vi "海流计数据编码.vi"() -> (3 "发送的信息":string)   [LabVIEW 2016, in "数据传输系统-03.lvlib"]
panel:
  out "层数 2":string
  out "层数参数位置 2":i32
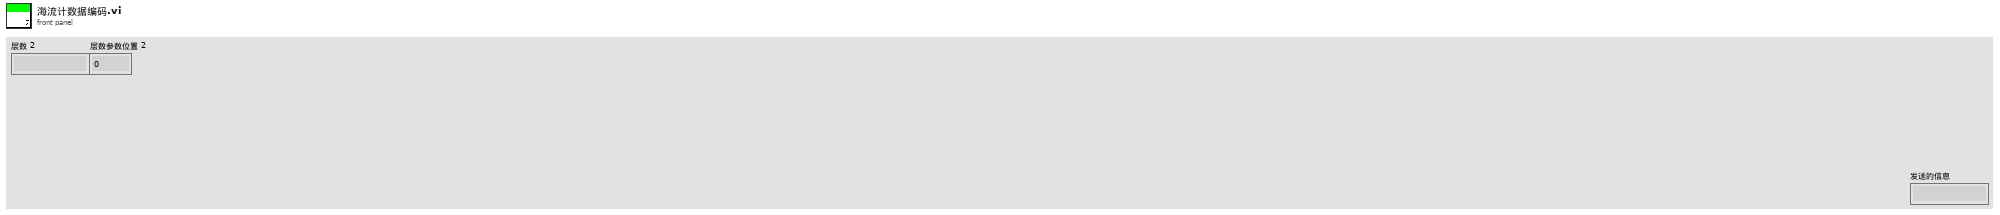
[diagram p1: front panel]
types:
  T1 = cluster{"CODMn":string, "CODCr":string, "DO":string, "铜":string, "PH":string, "氨氮":string, "比电导率":string, "水温":string, "COD":string, "浊度":string, "总氮":string, "总磷":string, "叶绿素a":string, "藻密度":string, "水位":string, "流速":string, "方向":string, "瞬时流量":string, "累积流量":string, "正累积流量":string, "负累积流量":string, "亚硝酸盐":string, "硫化物":string, "ORP":string, "铅":string, "镉":string, "锌":string, "镍":string, "锰":string, "汞":string, "气温":string, "气压":string, "风速":string, "风向":string, "空气温度":string, "相对湿度":string, "分钟雨量":string, "小时雨量":string, "日雨量":string, "累积雨量":string, "盐度":string, "磷酸盐":string, "硝氮":string, "氟化物":string, "挥发酚":string, "氯化物":string, "蓝绿藻":string, "余氯":string, "综合生物毒性":string, "艏向":string, "横摇":string, "纵摇":string, "分层标志":string, "层状态1":string, "层状态2":string, "水平平均流速":string, "流向":string, "北向流速分量":string, "东向流速分量":string, "垂直流速分量":string, "最大波高":string, "最大波周期":string, "1/10波高":string, "1/10波周期":string, "有效波高":string, "有效波周期":string, "平均波高":string, "平均波周期":string, "波向":string, "波个数":string, "水深":string, "X轴流速":string, "Y轴流速":string, "信号强度":string, "电压":string, "悬浮物":string}
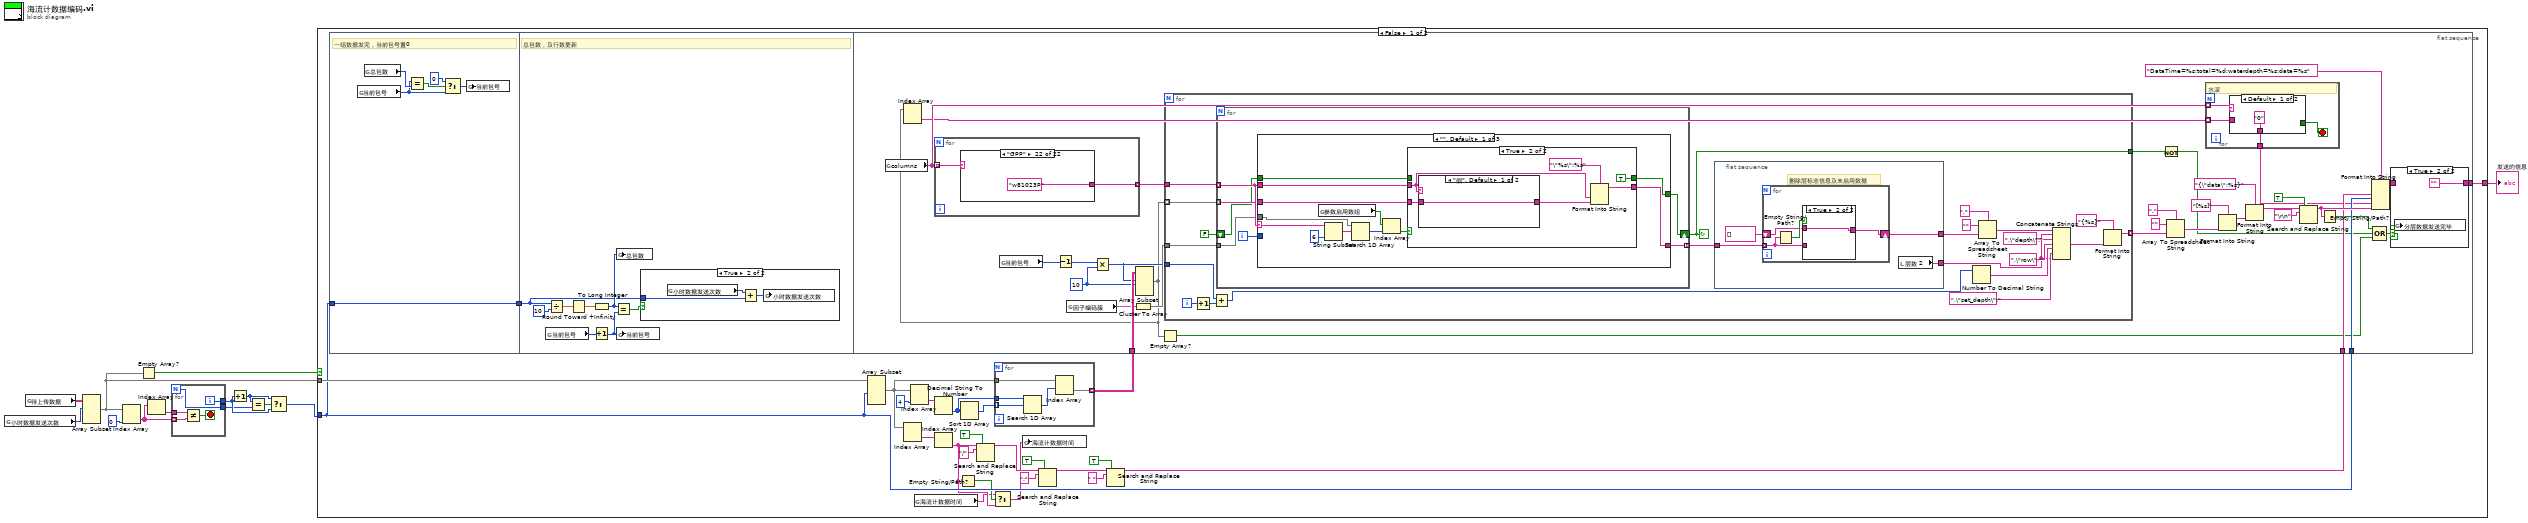
[diagram p0: block diagram]
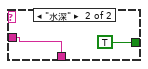
[diagram p3: hidden frame]
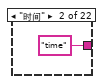
[diagram p6: hidden frame]
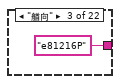
[diagram p7: hidden frame]
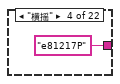
[diagram p8: hidden frame]
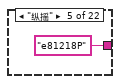
[diagram p9: hidden frame]
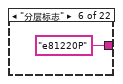
[diagram p10: hidden frame]
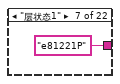
[diagram p11: hidden frame]
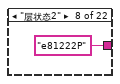
[diagram p12: hidden frame]
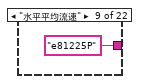
[diagram p13: hidden frame]
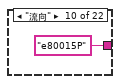
[diagram p14: hidden frame]
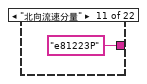
[diagram p15: hidden frame]
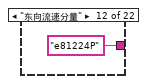
[diagram p16: hidden frame]
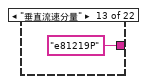
[diagram p17: hidden frame]
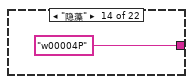
[diagram p18: hidden frame]
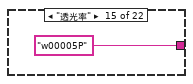
[diagram p19: hidden frame]
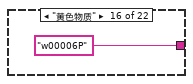
[diagram p20: hidden frame]
diagram:
  n1 = global read "全局 小时数据发送次数.vi" "小时数据发送次数"() -> (w13:i32)
  n2 = global read "全局 所有参数.vi" "待上传数据"() -> (w8:string[][])
  n3 = Array Subset(array=w8, index (row)=w13) -> (w6:string[][])  [unwired: 3 in]
  n4 = Index Array(array=w6, index (col)=0 ("禁用的索引 (列)")) -> (element=w11:string[])  [unwired: 1 in]
  n5 = Empty Array?(array=w6) -> (empty?=w7:bool)
  n6 = Index Array(array=w11) -> (element=w10:string)  [unwired: 1 in]
  n7 = for {
    N -> [w14]
    tunnel: w11 -> [w17] mode=indexing
    tunnel: w10 -> [w18]
    tunnel: [w15] -> w3
    tunnel: [w14] -> w2
    i -> [w15]
    stop <- w16 stop-if-true
    n8 = Not Equal?(x=w18, y=w17) -> (x != y?=w16:bool)
  }
  n9 = Increment(x=w3) -> (x+1=w4:i32)
  n10 = Equal?(x=w4, y=w2) -> (x = y?=w5:bool)
  n11 = Select(t=w4, s=w5, f=w3) -> (s? t:f=w1:i32)
  n12 = case shown="False" w7 {
    selector: w7 -> [_ w214]
    tunnel: w1 -> [w35 _]
    tunnel: w6 -> [w41 _]
    tunnel: [w19 _] -> w9
    frame False {
      n13 = flat-sequence {
        tunnel: w35 -> [w48]
        tunnel: [w48] -> w42
        tunnel: w42 -> [w54]
        tunnel: w37 -> [w97]
        tunnel: w35 -> [w77]
        tunnel: w20 -> [w76]
        tunnel: [w72] -> w19
        frame #0 {
          # "一组数据发完，当前包号置0"
          n14 = global read "全局 数据数组大小.vi" "当前包号"() -> (w51:i32)
          n15 = global read "全局 数据数组大小.vi" "总包数"() -> (w53:i32)
          n16 = Equal?(x=w51, y=w53) -> (x = y?=w52:bool)
          n17 = Select(t=0, s=w52, f=w51) -> (s? t:f=w49:i32)
          n18 = global write "全局 数据数组大小.vi" "当前包号"(w49) -> ()
        }
        frame #1 {
          # "总包数，及行数更新"
          n19 = global read "全局 数据数组大小.vi" "当前包号"() -> (w58:i32)
          n20 = Divide(x=w54, y=10) -> (x/y=w60:dbl)
          n21 = Round Toward +Infinity(x=w60) -> (ceil(x): smallest int >= x=w61:dbl)
          n22 = To Long Integer(number=w61) -> (32bit integer=w57:i32)
          n23 = Increment(x=w58) -> (x+1=w56:i32)
          n24 = Equal?(x=w57, y=w56) -> (x = y?=w55:bool)
          n25 = global write "全局 数据数组大小.vi" "总包数"(w57) -> ()
          n26 = global write "全局 数据数组大小.vi" "当前包号"(w56) -> ()
          n27 = case shown="True" w55 {
            tunnel: w54 -> [_ w63]
            frame False {
            }
            frame True {
              n28 = global read "全局 小时数据发送次数.vi" "小时数据发送次数"() -> (w64:i32)
              n29 = Add(x=w64, y=w63) -> (x+y=w62:i32)
              n30 = global write "全局 小时数据发送次数.vi" "小时数据发送次数"(w62) -> ()
            }
          }
        }
        frame #2 {
          w94 = 10 ("长度")
          n31 = global read "全局 所有参数.vi" "columns"() -> (w68:string[])
          n32 = for {
            tunnel: w68 -> [w109] mode=indexing
            tunnel: [w108] -> w91 mode=indexing
            n33 = case shown="\"GPP\"" w109 {
              tunnel: [_ "time" ("元素") "e81216P" "e81217P" "e81218P" "e81220P" "e81221P" "e81222P" "e81225P" "e80015P" "e81223P" "e81224P" "e81219P" "w00004P" "w00005P" "w00006P" "w00007P" "w01002P" "w01022P" "w81024P" "w81025P" "w81023P"] -> w108
              frame "", Default {
              }
              frame "时间" {
              }
              frame "艏向" {
              }
              frame "横摇" {
              }
              frame "纵摇" {
              }
              frame "分层标志" {
              }
              frame "层状态1" {
              }
              frame "层状态2" {
              }
              frame "水平平均流速" {
              }
              frame "流向" {
              }
              frame "北向流速分量" {
              }
              frame "东向流速分量" {
              }
              frame "垂直流速分量" {
              }
              frame "隐藻" {
              }
              frame "透光率" {
              }
              frame "黄色物质" {
              }
              frame "总藻" {
              }
              frame "盐度" {
              }
              frame "蓝绿藻" {
              }
              frame "Fv/Fm" {
              }
              frame "PAR" {
              }
              frame "GPP" {
              }
            }
          }
          n34 = global read "全局 数据数组大小.vi" "当前包号"() -> (w96:i32)
          n35 = Decrement(x=w96) -> (x-1=w95:i32)
          n36 = global read "断电保存全局.vi" "因子编码簇"() -> (w93:T1)
          n37 = Multiply(x=w95, y=w94) -> (x*y=w90:i32)
          n38 = Cluster To Array(cluster=w93) -> (array=w92:string[])
          n39 = Array Subset(array=w97, index (row)=w90, length (row)=w94) -> (w67:string[][])  [unwired: 2 in]
          n40 = Index Array(array=w67) -> (element=w66:string[])  [unwired: 2 in]
          n41 = Empty Array?(array=w67) -> (empty?=w69:bool)
          n42 = for {
            tunnel: w67 -> [w151] mode=indexing
            tunnel: w91 -> [w152]
            tunnel: [w147] -> w78 mode=indexing
            tunnel: w92 -> [w134]
            tunnel: [w132] -> w75
            tunnel: w90 -> [w131]
            i -> [w146]
            stop <- w132 continue-if-true
            n43 = Increment(x=w146) -> (x+1=w138:i32)
            n44 = Add(x=w131, y=w138) -> (x+y=w139:i32)
            n45 = for {
              tunnel: w152 -> [w170] mode=indexing
              tunnel: w151 -> [w169] mode=indexing
              tunnel: [w171] -> w137 mode=indexing
              tunnel: w134 -> [w167]
              shift-right: [w165] -> w132
              shift-left: FALSE -> [w166]
              i -> [w168]
              n46 = case shown="\"\", Default" w170 {
                selector: w170 -> [w175 _ _]
                tunnel: [w183 "" w212] -> w171
                tunnel: w170 -> [w182 w203 w211]
                tunnel: w169 -> [w181 w202 w207]
                tunnel: w168 -> [_ w201 _]
                tunnel: w167 -> [w180 _ _]
                tunnel: w166 -> [w176 w199 w205]
                tunnel: [w177 w199 w205] -> w165
                frame "", Default {
                  n47 = global read "断电保存全局.vi" "参数启用数组"() -> (w179:bool[])
                  n48 = String Subset(string=w175, length (rest)=6 ("长度（剩余）")) -> (substring=w173:string)  [unwired: 1 in]
                  n49 = Search 1D Array(1D array=w180, element=w173) -> (index of element=w178:i32)  [unwired: 1 in]
                  n50 = Index Array(array=w179, index=w178) -> (element=w172:bool)
                  n51 = case shown="True" w172 {
                    tunnel: ["" w190] -> w183
                    tunnel: w182 -> [_ w188]
                    tunnel: w181 -> [_ w187]
                    tunnel: [w184 TRUE] -> w177
                    tunnel: w176 -> [w184 _]
                    frame False {
                    }
                    frame True {
                      n52 = case shown="\"假\", Default" w188 {
                        tunnel: w187 -> [w192 w198]
                        tunnel: [w192 w193] -> w186
                        frame "假", Default {
                        }
                        frame "e81219P", "e81223P", "e81224P", "e81225P" {
                          n53 = Fract/Exp String To Number(string=w198) -> (number=w197:dbl)  [unwired: 3 in, 1 out]
                          n54 = Divide(x=w197, y=100.0) -> (x/y=w195:dbl)
                          n55 = Number To Fractional String(number=w195, precision (6)=i16 3 ("精度(6)")) -> (F-format string=w193:string)  [unwired: 2 in]
                        }
                      }
                      n56 = Format Into String(format string="\"%s\":%s" ("格式字符串"), w188, w186) -> (resulting string=w190:string)  [unwired: 2 in, 1 out]
                    }
                  }
                }
                frame "e81220P" {
                  n57 = Format Into String(format string="\"%s\":%s" ("格式字符串"), w203, w202) -> ()  [unwired: 2 in, 2 out]
                  "层数 2" <- w202
                  "层数参数位置 2" <- w201
                }
                frame "time" {
                  n58 = Search and Replace String(replace all?=TRUE ("替换全部？(F)"), input string=w207, search string="/" ("搜索字符串"), replace string="-" ("替换字符串(\"\")")) -> (result string=w206:string)  [unwired: 4 in, 3 out]
                  n59 = Format Into String(format string="\"%s\":\"%s\"" ("格式字符串"), w211, w206) -> (resulting string=w212:string)  [unwired: 2 in, 1 out]
                }
              }
            }
            n60 = flat-sequence {
              tunnel: w137 -> [w155]
              tunnel: [w156] -> w136
              tunnel: [w153] -> w135
              frame #0 {
                # "删除层标志信息及未启用数据"
                n61 = for {
                  tunnel: w155 -> [w157] mode=indexing
                  shift-right: [w158] -> w153
                  shift-left: string[] [] -> [w159]
                  n62 = Empty String/Path?(string/path=w157) -> (empty?=w160:bool)
                  n63 = case shown="True" w160 {
                    tunnel: [w161 w164] -> w158
                    tunnel: w159 -> [w163 w164]
                    tunnel: w157 -> [w162 _]
                    frame False {
                      n64 = Build Array (concatenate)(w163, w162) -> (w161:string[])
                    }
                    frame True {
                    }
                  }
                }
                n65 = local read "层数 2"() -> (w156:string)
              }
            }
            n66 = Number To Decimal String(number=w139) -> (decimal integer string=w143:string)  [unwired: 1 in]
            n67 = Array To Spreadsheet String(delimiter (Tab)="," ("分隔符(Tab)"), array=w135, 3:"" ("格式字符串")) -> (spreadsheet string=w141:string)
            n68 = Concatenate Strings(w141, ",\"depth\":", w136, ",\"row\":", w143, ",\"set_depth\":", w136) -> (w140:string)
            n69 = Format Into String(format string="{%s}" ("格式字符串"), w140) -> (resulting string=w147:string)  [unwired: 2 in, 1 out]
          }
          n70 = Not(x=w75) -> (.not. x?=w70:bool)
          n71 = Array To Spreadsheet String(delimiter (Tab)="," ("分隔符(Tab)"), array=w78, 3:"" ("格式字符串")) -> (spreadsheet string=w84:string)
          n72 = for {
            tunnel: w68 -> [w101] mode=indexing
            tunnel: w66 -> [w100] mode=indexing
            tunnel: [w98] -> w65
            stop <- w99 stop-if-true
            # "水深"
            n73 = case shown="Default" w101 {
              tunnel: w100 -> [_ w103]
              tunnel: [_ TRUE] -> w99
              tunnel: ["0" ("字符串") w103] -> w98
              frame Default {
              }
              frame "水深" {
              }
            }
          }
          n74 = Format Into String(format string="[%s]" ("格式字符串"), w84) -> (resulting string=w85:string)  [unwired: 2 in, 1 out]
          n75 = Format Into String(format string="{\"data\":%s}" ("格式字符串"), w85) -> (resulting string=w81:string)  [unwired: 2 in, 1 out]
          n76 = Search and Replace String(replace all?=TRUE ("替换全部？(F)"), input string=w81, search string="\r\n") -> (result string=w79:string)  [unwired: 5 in, 3 out]
          n77 = Empty String/Path?(string/path=w79) -> (empty?=w71:bool)
          n78 = Format Into String(format string="DataTime=%s;total=%d;waterdepth=%s;data=%s", w76, w77, w65, w79) -> (resulting string=w73:string)  [unwired: 2 in, 1 out]
          n79 = Compound Arithmetic op=OR ("复合运算")(w71, w70, w69) -> (w74:bool)
          n80 = case shown="True" w74 {
            selector: w74 -> [_ w106]
            tunnel: [w105 ""] -> w72
            tunnel: w73 -> [w105 _]
            frame False {
            }
            frame True {
              n81 = global write "全局 数据数组大小.vi" "分层数据发送完毕"(w106) -> ()
            }
          }
        }
      }
      n82 = Array Subset(array=w41, length (row)=w35) -> (w21:string[][])  [unwired: 3 in]
      n83 = Index Array(array=w21) -> (element=w34:string[])  [unwired: 2 in]
      n84 = Index Array(array=w21, index (col)=4 ("禁用的索引 (列)")) -> (element=w40:string[])  [unwired: 1 in]
      n85 = global read "全局 水样时间.vi" "海流计数据时间"() -> (w23:string)
      n86 = Decimal String To Number(string=w40) -> (number=w39:i32[])  [unwired: 2 in, 1 out]
      n87 = Index Array(array=w34) -> (element=w24:string)  [unwired: 1 in]
      n88 = Empty String/Path?(string/path=w24) -> (empty?=w25:bool)
      n89 = Sort 1D Array(array=w39) -> (sorted array=w38:i32[])
      n90 = Search and Replace String(replace all?=TRUE ("替换全部？(F)"), input string=w24, search string="/" ("替换字符串(\"\")")) -> (result string=w29:string)  [unwired: 5 in, 3 out]
      n91 = Select(t=w23, s=w25, f=w24) -> (s? t:f=w22:string)
      n92 = for {
        tunnel: w39 -> [w47]
        tunnel: w38 -> [w46] mode=indexing
        tunnel: w21 -> [w45]
        tunnel: [w43] -> w37 mode=indexing
        n93 = Search 1D Array(1D array=w47, element=w46) -> (index of element=w44:i32)  [unwired: 1 in]
        n94 = Index Array(array=w45, index (row)=w44) -> (element=w43:string[])  [unwired: 1 in]
      }
      n95 = global write "全局 水样时间.vi" "海流计数据时间"(w22) -> ()
      n96 = Search and Replace String(replace all?=TRUE ("替换全部？(F)"), input string=w29, search string=":" ("替换字符串(\"\")")) -> (result string=w26:string)  [unwired: 5 in, 3 out]
      n97 = Search and Replace String(replace all?=TRUE ("替换全部？(F)"), input string=w26, search string=" " ("替换字符串(\"\")")) -> (result string=w20:string)  [unwired: 5 in, 3 out]
    }
    frame True {
      n98 = global write "全局 数据数组大小.vi" "分层数据发送完毕"(w214) -> ()
    }
  }
  "发送的信息" <- w9
